vi "Miniquads.SetVerticalVoltage.vi"(0 "i ref in":refnum<vi>, 2 "VerticalVoltage":dbl, 3 "ms timeout (10000)":i32=10000, 5 "error in (no error)":errorcluster) -> (14 "i ref out":refnum<vi>, 17 "timed out":bool, 19 "error out":errorcluster)   [LabVIEW 2014, in "Miniquads.lvlib"]
doc: "Sets the VerticalVoltage."
uses:
  Miniquads.lvlib
  CSCore/CSApplicationBaseClasses/DeviceBase/DeviceBase.lvlib
  CSlibraries-extern/DimLVEvent/LVDimInterface/LVDimInterface.lvlib
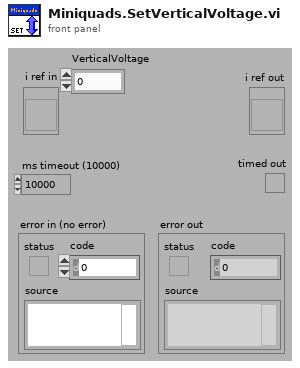
[diagram p1: front panel]
types:
  T1 = typedef "Miniquads.lvlib/Miniquads.i attribute.ctl" = cluster{"ObjectsInitialized":bool, "ObjectsLoaded":string[], "nomValues":T2, "actValues":T2}
  T2 = typedef "Miniquads.lvlib/Miniquads.voltages.ctl" = cluster{"FocusVoltage":dbl, "HorizontalVoltage":dbl, "VerticalVoltage":dbl, "serviceIDs":cluster{"FocusVoltageID":i32, "HorizontalVoltageID":i32, "VerticalVoltageID":i32}}
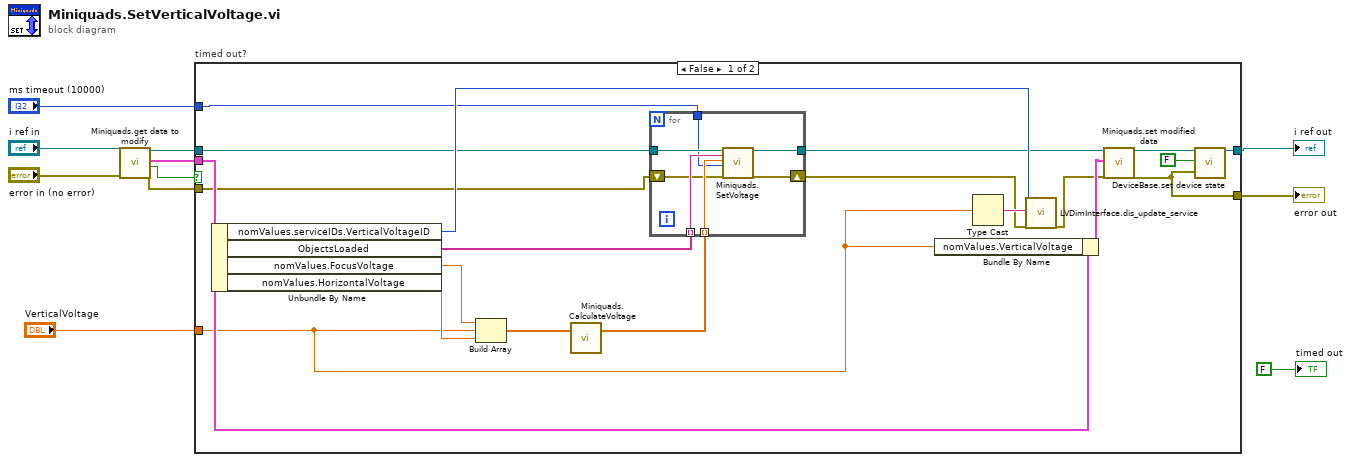
[diagram p0: block diagram]
diagram:
  n1 = call "Miniquads.get data to modify.vi"("i ref in"="i ref in", "error in (no error)"="error in (no error)") -> ("i ref out"=w5:refnum<vi>, "i attribute"=w1:T1, "timed out"=w3:bool, "error out"=w2:errorcluster)  [unwired: 14 in]
  n2 = case "timed out?" shown="False" w3 {
    tunnel: w5 -> [w22 w40]
    tunnel: [w28 w40] -> w11
    tunnel: [w29 w39] -> w9
    tunnel: "ms timeout (10000)" -> [w19 _]
    tunnel: "VerticalVoltage" -> [w12 _]
    tunnel: w2 -> [w18 w39]
    tunnel: w1 -> [w26 _]
    frame False {
      n3 = Unbundle By Name(w26) -> ("nomValues.serviceIDs.VerticalVoltageID"=w24:i32, "ObjectsLoaded"=w21:string[], "nomValues.FocusVoltage"=w14:dbl, "nomValues.HorizontalVoltage"=w13:dbl)
      n4 = Build Array(w14, w12, w13) -> (w15:dbl[])
      n5 = call "Miniquads.CalculateVoltage.vi"("Miniquad Voltages"=w15) -> ("ChannelVoltages"=w20:dbl[])  [unwired: 18 in]
      n6 = for {
        tunnel: w22 -> [w38]
        tunnel: [w37] -> w16
        tunnel: w21 -> [w36] mode=indexing
        tunnel: w20 -> [w35] mode=indexing
        tunnel: w19 -> [w34]
        shift-right: [w33] -> w17
        shift-left: w18 -> [w32]
        n7 = call "Miniquads.SetVoltage.vi"("i ref in"=w38, "Object"=w36, "SetVoltage"=w35, "ms timeout (10000)"=w34, "error in (no error)"=w32) -> ("i ref out"=w37:refnum<vi>, "error out"=w33:errorcluster)  [unwired: 12 in, 1 out]
      }
      n8 = Bundle By Name(cluster=w26, "nomValues.VerticalVoltage"=w12) -> (w27:T1)
      n9 = Type Cast(x=w12) -> (*(type *) &x=w25:string)  [unwired: 1 in]
      n10 = call "LVDimInterface.dis_update_service.vi"("my_serviceID"=w24, "data"=w25, "error in (no error)"=w17) -> ("error out"=w23:errorcluster)  [unwired: 14 in, 2 out]
      n11 = call "Miniquads.set modified data.vi"("i ref in"=w16, "i attribute"=w27, "error in (no error)"=w23) -> ("i ref out"=w31:refnum<vi>, "error out"=w29:errorcluster)  [unwired: 15 in]
      n12 = call "DeviceBase.set device state.vi"("i ref in"=w31, "implicit"=FALSE, "device error"=w29) -> ("i ref out"=w28:refnum<vi>)  [unwired: 14 in, 2 out]
    }
    frame True {
    }
  }
  "error out" <- w9
  "i ref out" <- w11
  "timed out" <- FALSE ("timed out")
